vi "LS330_Set_Range.vi"(7 "error in":errorcluster, 8 "Range":T1, 9 "Heater":string(combo)="1", 10 "VISA resource name":refnum<visa-resource-name>) -> (0 "error out":errorcluster, 3 "VISA resource name out":refnum<visa-resource-name>)   [LabVIEW 2021]
uses:
  Heater_Range.ctl
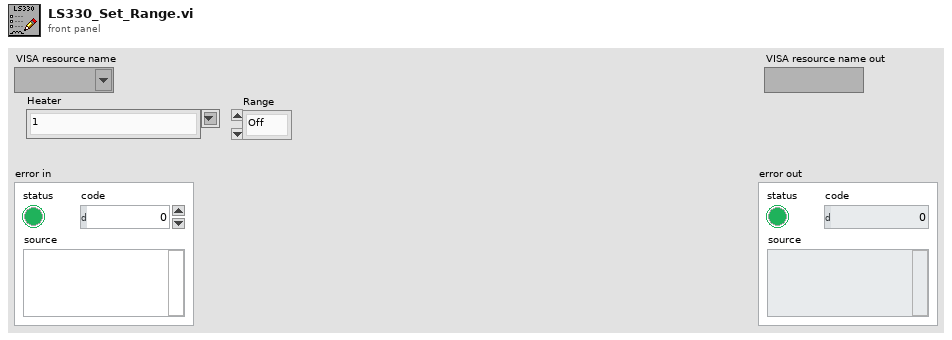
[diagram p1: front panel]
types:
  T1 = typedef "Heater_Range.ctl" = enum16{"Off", "Low", "Medium", "High"}
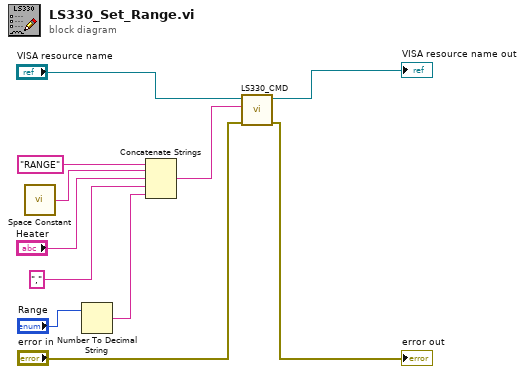
[diagram p0: block diagram]
diagram:
  n1 = call <vilib>:"Space Constant.vi"() -> ("String"=w9:string)
  n2 = Number To Decimal String(number="Range") -> (decimal integer string=w1:string)  [unwired: 1 in]
  n3 = Concatenate Strings("RANGE" ("string"), w9, "Heater", ",", w1) -> (w7:string)
  n4 = call "LS330_CMD.vi"("error in"="error in", "CMD"=w7, "VISA resource name"="VISA resource name") -> ("error out"=→"error out":errorcluster, "VISA resource name out"=→"VISA resource name out":refnum<visa-resource-name>)  [unwired: 7 in]
